vi "Actor Core.vi"(8 "error in":errorcluster, 11 "Test Node Charm View in":refnum<class "Test Node Charm View.lvclass">) -> (0 "error out":errorcluster, 3 "Actor out":refnum<class "Actor.lvclass">)   [LabVIEW 2013, in "Test Node Charm View.lvlib" / "Test Node Charm View.lvclass"]
doc: "(<B>Filename</B>: Actor Framework.lvlib:Actor.lvclass:Actor Core.vi)\n\nReceives messages to the actor, reacts to them, and initiates any error handling that may shut the actor down.\n\nDescendant classes may override this VI to append parallel tasks for the actor to complete while it handles messages. Overrides use the Call Parent Method node."
uses:
  Test Node Charm View.lvclass
  <vilib>/ActorFramework/Actor/Actor.lvclass
  <vilib>/ActorFramework/Actor/Actor.lvclass/Actor.ctl
  <vilib>/ActorFrameworkMVC/View Actor/View Actor.lvclass
  <vilib>/ActorFrameworkMVC/UI Controller Messages/Move Splitter Msg/Move Splitter Msg.lvclass/Move Splitter Msg.ctl
  <vilib>/ActorFramework/Message Enqueuer/Message Enqueuer.lvclass/Message Enqueuer.ctl
  <vilib>/ActorFramework/Message Enqueuer/Enqueue.vi
  <vilib>/ActorFramework/Message Priority Queue/Priority Enqueue.vi
  <vilib>/ActorFrameworkMVC/UI Controller Messages/Move Splitter Msg/Move Splitter Msg.lvclass
  Models/Test Node Model Messages/Remove Test Node Msg/Remove Test Node Msg.lvclass
  <vilib>/ActorFrameworkMVC/UI Controller Messages/Get Model Actor Enqueuer Msg/Get Model Actor Enqueuer Msg.lvclass
panel:
  in  "Test Channel":bool
  in  "Remove":bool
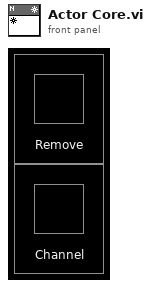
[diagram p1: front panel]
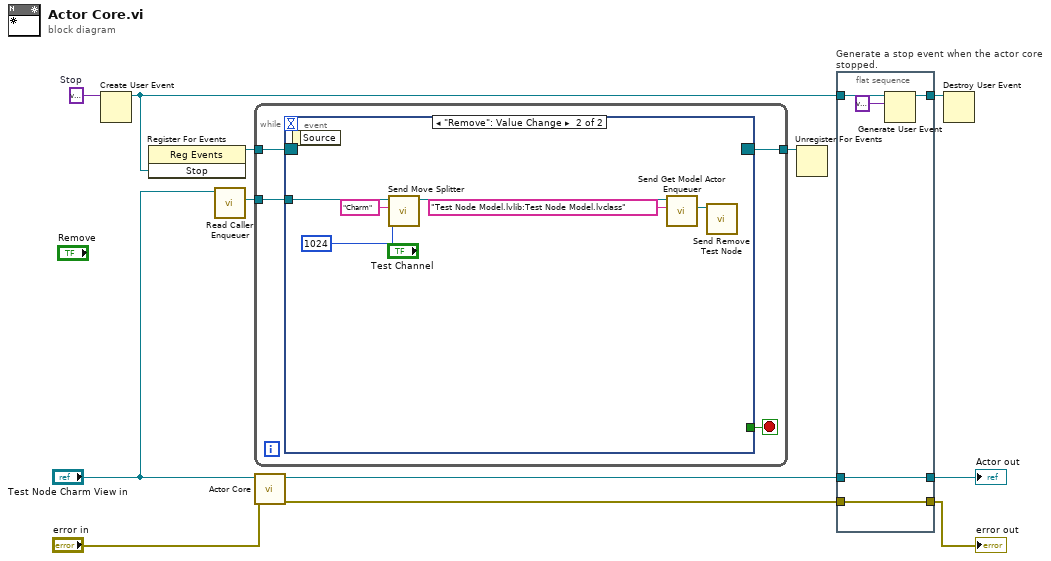
[diagram p0: block diagram]
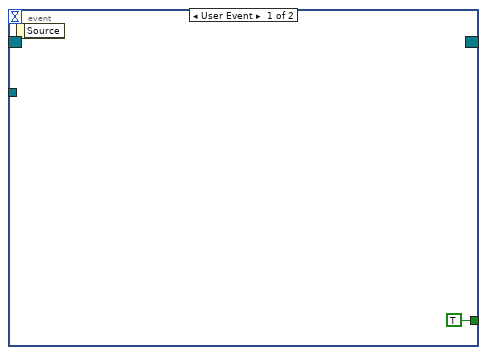
[diagram p2: hidden frame]
diagram:
  w12 = variant  # Stop
  n1 = Create User Event(user event datatype=w12) -> (user event=w4:refnum<user-event>)  [unwired: 1 in, 1 out]
  n2 = register-events(w4) -> (reference out=w5:refnum<event-registration>)  [unwired: 2 in, 1 out]
  n3 = call <vilib>:"Read Caller Enqueuer.vi"("Actor"="Test Node Charm View in") -> ("Caller Enqueuer"=w1:refnum<class "Message Enqueuer.lvclass">)  [unwired: 10 in]
  n4 = while {
    tunnel: [w16] -> w3
    tunnel: w5 -> [w14]
    tunnel: w1 -> [w13]
    stop <- w15 stop-if-true
    n5 = event shown="[1] \"Remove\": Value Change" {
      selector: w14 -> [_ _]
      dyn-events: [_ _] -> w16
      timeout: _ -> [_ _]
      tunnel: [TRUE _] -> w15
      tunnel: w13 -> [_ w18]
      event User Event {
        n6 = event-data() -> ()  [unwired: 1 in, 1 out]
      }
      event "Remove": Value Change {
        n7 = event-data() -> ()  [unwired: 1 in, 1 out]
        n8 = call <vilib>:"Send Move Splitter.vi"("Splitter Position"=1024, "Splitter Name"="Charm", "Message Enqueuer"=w18) -> ("Message Enqueuer out"=w21:refnum<class "Message Enqueuer.lvclass">)  [unwired: 7 in, 1 out]
        n9 = call <vilib>:"Send Get Model Actor Enqueuer.vi"("Model Name"="Test Node Model.lvlib:Test Node Model.lvclass", "Message Enqueuer in"=w21) -> ("Reply"=w22:refnum<class "Message Enqueuer.lvclass">)  [unwired: 6 in, 3 out]
        n10 = call "Send Remove Test Node.vi"("Message Enqueuer"=w22) -> ()  [unwired: 9 in, 2 out]
      }
    }
  }
  n11 = call-parent "Actor Core.vi"("error in"="error in", "View Actor in"="Test Node Charm View in") -> ("error out"=w8:errorcluster, "Actor out"=w9:refnum<class "Actor.lvclass">)  [unwired: 8 in]
  n12 = Unregister For Events(event registration refnum=w3) -> ()  [unwired: 1 in, 1 out]
  n13 = flat-sequence "Generate a stop event when the actor core stopped." {
    tunnel: w4 -> [w28]
    tunnel: [w26] -> w11
    tunnel: w9 -> [w25]
    tunnel: w8 -> [w24]
    tunnel: [w25] -> w7
    tunnel: [w24] -> w6
    frame #0 {
      n14 = Generate User Event(user event=w28, event data cluster=variant ("event data")) -> (user event out=w26:refnum<user-event>)  [unwired: 2 in, 1 out]
    }
  }
  n15 = Destroy User Event(user event=w11) -> ()  [unwired: 1 in, 1 out]
  "error out" <- w6
  "Actor out" <- w7
